vi "AdvancedSerial.vi"(8 "error in (no error)":errorcluster, 9 "All Files in Dir":path[](array[path]), 10 "new name":string, 11 "Python in":T1) -> (0 "error out":errorcluster, 3 "Python out":T1)   [LabVIEW 2022 SP3]
uses:
  PythonCtrl.ctl
  Processors.ctl
  <vilib>/Utility/error.llb/Trim Whitespace One-Sided.vi
panel:
  in  "Done":bool
  out "saved":string[](array[string])
  out "codes":string[](array[string])
  in  "Files to copy over":i32(listbox)
  out "progress":u8(slide) scale=0.0..100.0
  in  "Stop":bool
  in  "Port in":string
  in  "Python version":string="3.9"
  out "fileName":string="test.py"
  out "Code":string="import os\nimport time\n\ntime.sleep(1)\nos.listdir()"
  out "chosen":string
  out "file saved":string
  out "possible ports":string[](array[string])
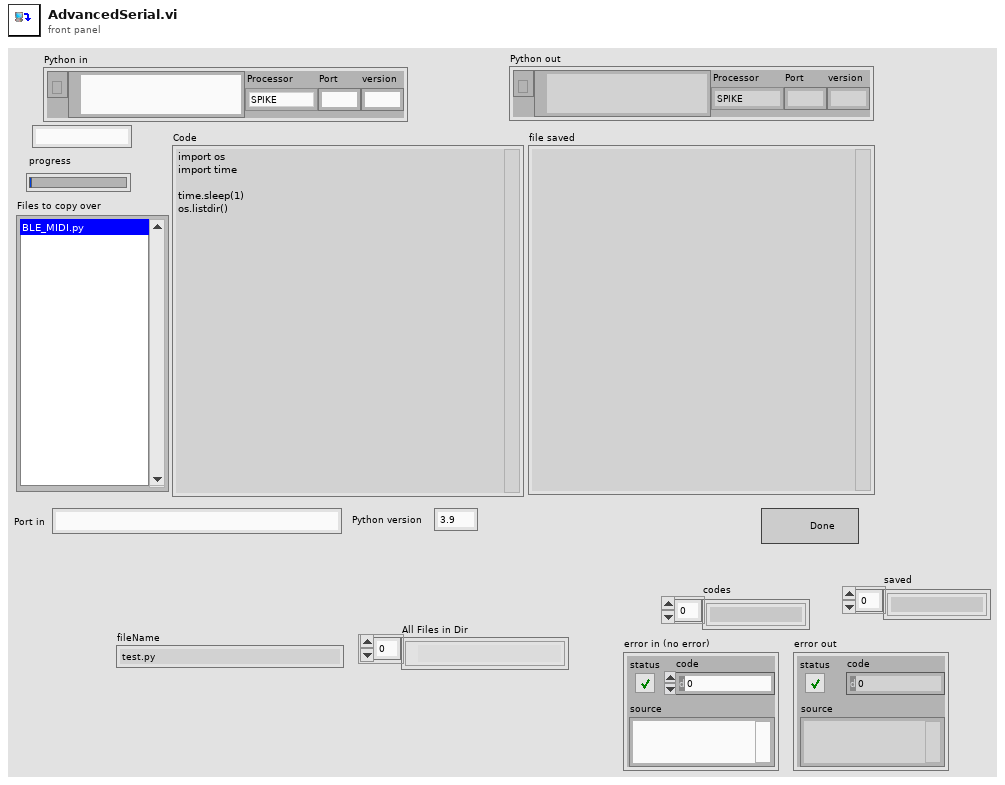
[diagram p1: front panel]
types:
  T1 = typedef "PythonCtrl.ctl" = cluster{"session":refnum<k35>, "PyPath":path, "Processor":T2, "Port":string, "version":string}
  T2 = typedef "Processors.ctl" = enum16{"SPIKE", "Pi", "Pi_ssh", "OpenMV", "Dunio"}
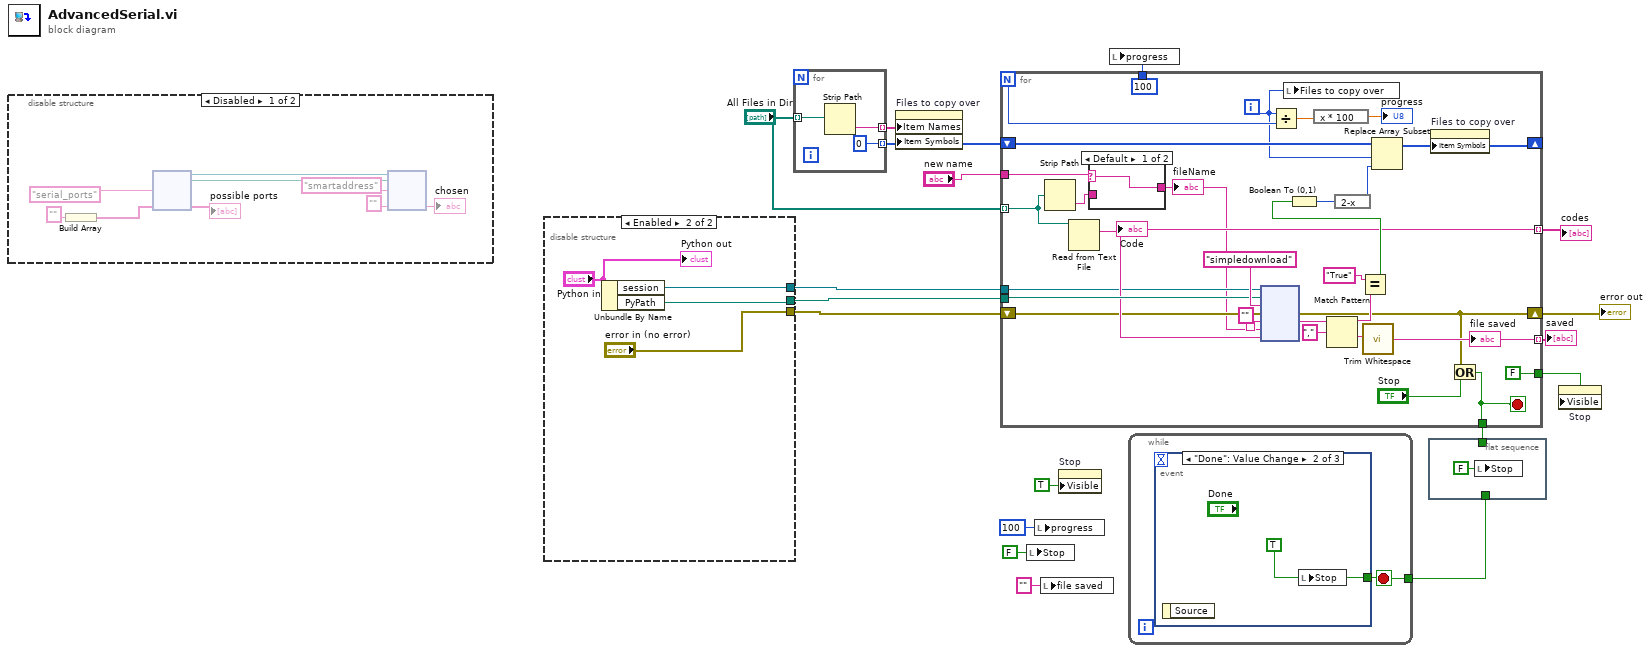
[diagram p0: block diagram]
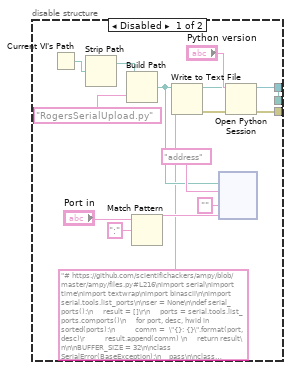
[diagram p2: hidden frame]
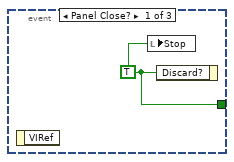
[diagram p3: hidden frame]
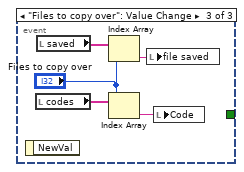
[diagram p4: hidden frame]
diagram:
  n1 = disable-structure shown="Disabled" {
    frame Disabled {
      n2 = Build Array("" ("function name")) -> (w28:string[])
      n3 = node(w19, "serial_ports" ("function name"), w28) -> (w20:refnum<k35>, w23:refnum<k35>, w29:errorcluster, →"possible ports":string[])  [unwired: 3 out]
      n4 = node(w23, "smartaddress" ("function name"), "" ("function name")) -> (w19:path, →"chosen":string)  [unwired: 1 in, 4 out]
    }
    frame Enabled {
    }
  }
  n5 = disable-structure shown="Enabled" {
    disable-tunnel: [w38 w47] -> w18
    disable-tunnel: [w37 "error in (no error)"] -> w17
    disable-tunnel: [w31 w46] -> w16
    frame Disabled {
      n6 = Current VI's Path() -> (path=w41:path)
      n7 = Strip Path(path=w41) -> (stripped path=w42:path)  [unwired: 1 out]
      n8 = Build Path(base path=w42, name or relative path="RogersSerialUpload.py") -> (appended path=w31:path)
      n9 = Match Pattern(string="Port in", regular expression=":") -> (before substring=w32:string)  [unwired: 1 in, 3 out]
      n10 = Write to Text File(file (use dialog)=w31, text="# https://github.com/scientifichackers/ampy/blob/master/ampy/files.py#L216\nimport serial\nimport time\nimport textwrap\nimport binascii\n\nimport serial.tools.list_ports\n\nser = None\n\ndef serial_ports():\n     result = []\r\n     ports = serial.tools.list_ports.comports()\n     for port, desc, hwid in sorted(ports):\n          comm =  \"{}: {}\".format(port, desc)\r          result.append(comm) \n     return result\n\n\nBUFFER_SIZE = 32\n\nclass SerialError(BaseException):\n    pass\n\nclass campy():\n    def __init__(self, device = None, verbose = False):\n        self.device = device\n        self.serial = None\n        self.verbose = verbose\n\n    def address(self, device):\n        self.device=device\n        \n    def printIt(self, payload):\n        if self.verbose:\n            print(payload)\n        \n    def open_serial(self):\n        try:\n            self.serial = serial.Serial(self.device, baudrate=115200, interCharTimeout=1, timeout = 0)\n        except Exception as e:\n            print(e)\n            \n    def close_serial(self):\n        self.serial.close()\n\n    def flush(self):\n        n = self.serial.inWaiting()\n        while n > 0:\n            self.serial.read(n)\n            n = self.serial.inWaiting()\n\n    def read_until(self, min_len, ending, timeout = 10):\n        data = self.serial.read(min_len)\n        timeout_count = 0\n        while True:\n            #print(data)\n            if data.endswith(ending):\n                break\n            elif self.serial.inWaiting() > 0:\n                new_data = self.serial.read(1)\n                data = data + new_data\n                timeout_count = 0\n            else:\n                timeout_count += 1\n                if timeout is not None and timeout_count >= 1 * timeout: #used to be 100 *\n                    self.printIt('timeout')\n                    self.printIt(ending)\n                    self.printIt(data)\n                    break\n                time.sleep(0.01)\n        return data\n\n    def send_get(self, payload, expected, tries = 1):\n        for retry in range(0, tries): \n            self.serial.write(payload) \n            data = self.read_until(1, expected)\n            if data.endswith(expected):\n                self.printIt('Read: ' + repr(data))\n                return True\n        raise SerialError('no raw mode')\n  \n    def run_line(self, command):\n        if isinstance(command, bytes): command_bytes = command\n        else: command_bytes = bytes(command, encoding='utf8')\n        self.flush()\n        #self.read_until(1, b'>')\n        self.printIt('Sending: '+ repr(command))\n        for i in range(0, len(command_bytes), 256):\n            self.serial.write(command_bytes[i:min(i + 256, len(command_bytes))])\n            time.sleep(0.01)\n        self.send_get(b'\\x04',b'OK',1)\n                    \n    def go_raw(self):\n        self.serial.write(b'\\r\\x03')\n        time.sleep(0.1)\n        self.serial.write(b'\\x03')\n        time.sleep(0.1)\n        self.flush()\n\n        self.send_get(b'\\r\\x01', b'raw REPL; CTRL-B to exit\\r\\n>', 5)\n        self.send_get(b'\\x04', b'soft reboot\\r\\n', 1)\n        time.sleep(0.5)\n        self.serial.write(b'\\x03')\n        time.sleep(0.1) \n        self.send_get(b'\\x03', b'raw REPL; CTRL-B to exit\\r\\n', 1)\n\n    def close_raw(self):\n        self.serial.write(b'\\r\\x02') # ctrl-B: enter friendly REPL\n        \n    def send_code(self, filename, data):\n       self.run_line(\"f = open('%s', 'wb')\"%(filename))\n        size = len(data)\n        # Loop through and write a buffer size chunk of data at a time.\n        for i in range(0, size, BUFFER_SIZE):\n            chunk_size = min(BUFFER_SIZE, size - i)\n            chunk = repr(data[i : i + chunk_size])\n            # Make sure to send explicit byte strings (handles python 2 compatibility).\n            if not chunk.startswith(\"b\"):\n                chunk = \"b\" + chunk\n            self.run_line(\"f.write(%s)\"%(chunk))\n        self.run_line(\"f.close()\")\n\n    def download(self, filename, data):\n        self.open_serial()\n        self.go_raw()\n        self.send_code()\n        self.close_raw()\n        self.close_serial()\n        payload =  fred.upload(filename).decode()\n        return (data == payload), payload\n        \n    def upload(self, filename):\n        command = \"\"\"\n            import sys\n            import ubinascii\n            with open('%s', 'rb') as infile:\n                while True:\n                    result = infile.read(%d)\n                    if result == b'':\n                        break\n                    len = sys.stdout.write(ubinascii.hexlify(result))\n        \"\"\" % (filename, BUFFER_SIZE)\n        \n        self.open_serial()\n        self.go_raw()\n        try:\n            self.run_line(textwrap.dedent(command))\n            out = self.read_until(1, b'\\x04')\n            self.printIt(out)\n        except SerialError as ex:\n            # Check if this is an OSError #2, i.e. file doesn't exist and\n            # rethrow it as something more descriptive.\n            try:\n                message = ex.args[2].decode(\"utf-8\")\n                if message.find(\"OSError\") != -1 and message.find(\"2\") != -1:\n                    raise RuntimeError(\"No such file: {0}\".format(filename))\n                else:\n                    raise ex\n            except UnicodeDecodeError:\n                raise ex\n        self.close_raw()\n        self.close_serial()\n        out = out[:-1]\n        return binascii.unhexlify(out)\n\nfred=campy('COM3')\n\ndef address(device):\n    fred.address(device)\n\ndef smartaddress():\n    device = '/dev/cu.usbmodem1101'\n    ports = serial_ports()\n    for port in ports:\n        if 'cu.usb' in port:\n            device = port.split(':')[0]\n            fred.device = device\n            break\n    return device\n\ndef download(file, code):\n    s, p = fred.download(file,code)\n    return str(s) +','+ p\n\ndef upload(file):\n    return  fred.upload(file).decode()\n\n") -> (error out=w39:errorcluster)  [unwired: 2 in, 2 out]
      n11 = node(w31, "address" ("function name"), "" ("function name"), w32) -> ()  [unwired: 4 in, 4 out]
      n12 = Open Python Session(python version="Python version", 3:w39) -> (session out=w38:refnum<k35>, error out=w37:errorcluster)  [unwired: 1 in]
    }
    frame Enabled {
      n13 = Unbundle By Name("Python in") -> ("session"=w47:refnum<k35>, "PyPath"=w46:path)
      "Python out" <- "Python in"
    }
  }
  n14 = for {
    tunnel: "All Files in Dir" -> [w50] mode=indexing
    tunnel: [w49] -> w9 mode=indexing
    tunnel: [0] -> w8 mode=indexing
    n15 = Strip Path(path=w50) -> (name=w49:string)  [unwired: 1 out]
  }
  n16 = property on="Files to copy over" class="LstBox (strict)"("Item Names"=w9, "Item Symbols"=w8) -> ()  [unwired: 2 in, 2 out]
  n17 = for {
    N -> [w69]
    tunnel: "All Files in Dir" -> [w80] mode=indexing
    tunnel: w18 -> [w55]
    tunnel: w16 -> [w72]
    tunnel: [100] -> w15
    tunnel: [w57] -> w12
    shift-right: [w63] -> _
    shift-left: w8 -> [w67]
    tunnel: [w62] -> w7 mode=indexing
    tunnel: [w61] -> w6 mode=indexing
    tunnel: [FALSE ("Stop")] -> w4
    shift-right: [w54] -> w3
    shift-left: w17 -> [w56]
    tunnel: "new name" -> [w53]
    i -> [w60]
    stop <- w57 stop-if-true
    n18 = Strip Path(path=w80) -> (name=w51:string)  [unwired: 1 out]
    n19 = Read from Text File(file (use dialog)=w80) -> (text=w61:string)  [unwired: 3 in, 3 out]
    "Code" <- w61
    n20 = case shown="Default" w53 {
      selector: w53 -> [w81 _]
      tunnel: [w81 w82] -> w52
      tunnel: w51 -> [_ w82]
      frame Default {
      }
      frame "" {
      }
    }
    "fileName" <- w52
    n21 = node(w55, w72, "simpledownload" ("function name"), w56, "" ("function name"), w52, w61) -> (w54:errorcluster, w77:string)  [unwired: 2 in, 3 out]
    n22 = Divide(x=w60, y=w69) -> (x/y=w71:dbl)
    n23 = local write "Files to copy over"(w60) -> ()
    n24 = expression code="x * 100"(w71) -> (→"progress":dbl)
    n25 = Match Pattern(string=w77, regular expression=",") -> (before substring=w79:string, after substring=w78:string)  [unwired: 1 in, 2 out]
    n26 = Equal?(x="True" ("regular expression"), y=w79) -> (x = y?=w66:bool)
    n27 = Boolean To (0,1)(Boolean=w66) -> (0, 1=w65:i16)
    n28 = expression code="2-x"(w65) -> (w64:i16)
    n29 = call <vilib>:"Trim Whitespace.vi"("string"=w78) -> ("trimmed string"=w62:string)  [unwired: 1 in]
    "file saved" <- w62
    n30 = Replace Array Subset(array=w67, new element=w64, index=w60) -> (w63:i32[])
    n31 = property on="Files to copy over" class="LstBox (strict)"("Item Symbols"=w63) -> ()  [unwired: 2 in, 2 out]
    n32 = Or(x=w54, y="Stop") -> (x .or. y?=w57:bool)
  }
  "codes" <- w6
  "saved" <- w7
  "error out" <- w3
  n33 = local write "Stop"(FALSE ("Stop")) -> ()
  n34 = local write "progress"(u8 100 ("progress")) -> ()
  n35 = local write "file saved"("" ("file saved")) -> ()
  n36 = property on="Stop" class="Bool (strict)"("Visible"=TRUE) -> ()  [unwired: 2 in, 2 out]
  n37 = local write "progress"(w15) -> ()
  n38 = while {
    tunnel: [w83] -> w11
    stop <- w83 stop-if-true
    n39 = event shown="[1] \"Done\": Value Change" {
      selector: _ -> [_ _ _]
      dyn-events: _ -> [_ _ _]
      timeout: _ -> [_ _ _]
      tunnel: [w84 w85 _] -> w83
      event Panel Close? {
        w84 = TRUE ("Discard?")
        n40 = event-data() -> ()  [unwired: 1 in, 1 out]
        n41 = local write "Stop"(w84) -> ()
        n42 = event-data("Discard?"=w84) -> ()  [unwired: 1 in, 1 out]
      }
      event "Done": Value Change {
        w85 = TRUE ("Discard?")
        n43 = event-data() -> ()  [unwired: 1 in, 1 out]
        n44 = local write "Stop"(w85) -> ()
      }
      event "Files to copy over": Value Change {
        n45 = event-data() -> ()  [unwired: 1 in, 1 out]
        n46 = local read "codes"() -> (w89:string[])
        n47 = local read "saved"() -> (w90:string[])
        n48 = Index Array(array=w90, index="Files to copy over") -> (element=w87:string)
        n49 = Index Array(array=w89, index="Files to copy over") -> (element=w88:string)
        n50 = local write "file saved"(w87) -> ()
        n51 = local write "Code"(w88) -> ()
      }
    }
  }
  n52 = flat-sequence {
    tunnel: w12 -> [_]
    tunnel: w11 -> [_]
    frame #0 {
      n53 = local write "Stop"(FALSE ("Stop")) -> ()
    }
  }
  n54 = property on="Stop" class="Bool (strict)"("Visible"=w4) -> ()  [unwired: 2 in, 2 out]
